vi "LSX Get BPZ Trackball Factor.vi"(8 "error in (no error)":errorcluster, 10 "pdAValue":dbl, 11 "lLSID":i32) -> (0 "error out":errorcluster, 2 "pdAValue out":dbl, 3 "function return":i32)   [LabVIEW 2018, in "Tango.lvlib"]
doc: "TANGOAPI int TANGOCALL LSX_GetBPZTrackballFactor (int lLSID, double *pdAValue);"
uses:
  <userlib>/Tango/Tango.lvlib
  <userlib>/Tango/Tango_DLL.dll
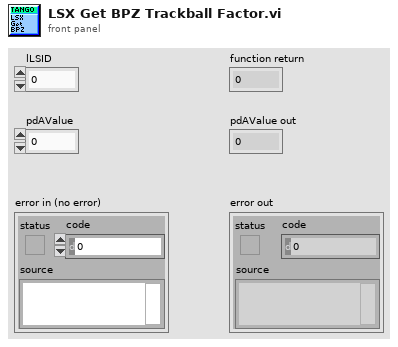
[diagram p1: front panel]
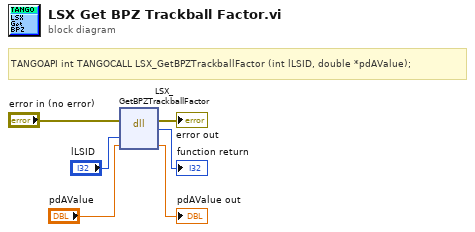
[diagram p0: block diagram]
diagram:
  # "TANGOAPI int TANGOCALL LSX_GetBPZTrackballFactor (int lLSID, double *pdAValue);"
  n1 = dll-call lib="C:/Program Files (x86)/National Instruments/LabVIEW 2018/user.lib/Tango/Tango_DLL.*" fn="LSX_GetBPZTrackballFactor"(error in="error in (no error)", "lLSID"="lLSID", "pdAValue"="pdAValue") -> (error out=→"error out":errorcluster, →"function return":i32, "pdAValue"=→"pdAValue out":dbl)  [unwired: 3 in, 1 out]
